vi "main_track.vi"(7 "camera notifier":refnum<notifier>, 8 "error in (no error)":errorcluster, 9 "tracking notifier in":refnum<notifier>, 10 "Median Filter Image":T2, 11 "Session In":T1) -> (0 "error out":errorcluster)   [LabVIEW 2019]
uses:
  <vilib>/vision/Image Controls.llb/IMAQ Image.ctl
  <vilib>/userdefined/High Color/IMAQdx.ctl
  CompletedTracksFunctionalGlobalOperations.ctl
  ActiveTracksFunctionalGlobalOperations.ctl
  <vilib>/vision/driver/IMAQdx.llb/IMAQdx Buffer Number Mode.ctl
  WormTrackSnippetCluster.ctl
  TrackTerminationReasonEnum.ctl
  <vilib>/Utility/error.llb/DialogType.ctl
  euclidean_distance_single.vi
  ParametersGlobal.vi
  DebugGlobal.vi
  StimulusObject.lvclass
  <vilib>/vision/NI_Vision_Development_Module.lvlib
  <vilib>/vision/driver/NI_Vision_Acquisition_Software.lvlib
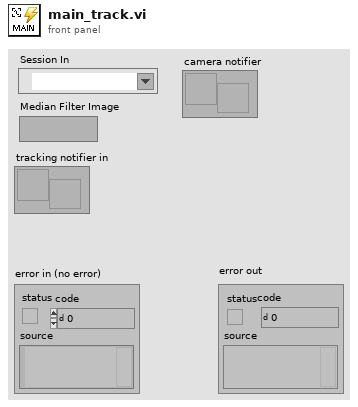
[diagram p1: front panel]
types:
  T1 = typedef "IMAQdx.ctl" = refnum<k21>
  T2 = typedef "IMAQ Image.ctl" = refnum<image>
  T3 = typedef "Particle Parameters" = i32
  T4 = cluster{"Measurement Parameter":T3, "Range Lower Value":dbl, "Range Upper Value":dbl, "Range":bool, "Measurement Type":bool}
  T5 = typedef "Image Type" = u32
  T6 = cluster{"Measurement Parameter":T3, "Range Lower Value":dbl, "Range Upper Value":dbl, "Range":bool, "Measurement Type":bool}[]
  T7 = typedef "NI_Vision_Acquisition_Software.lvlib/IMAQdx Buffer Number Mode.ctl" = enum32{"Next", "Last", "Buffer Number", "Every", "Last New"}
  T8 = typedef "ActiveTracksFunctionalGlobalOperations.ctl" = enum16{"Initialize", "ReadFullTrackGivenWormIndex", "WriteFullTrack", "ReadTrackSnippets", "WriteTrackGivenSnippets", "ReadStimulusSnippets", "StartNewTracksGivenSnippets", "EndTracksGivenSnippets", "WriteStimulusObjectGivenWormIndex", "CompleteAllActiveTracks", "ReturnAllActiveTrackIndecies"}
  T9 = typedef "CompletedTracksFunctionalGlobalOperations.ctl" = enum16{"Initialize", "ReturnAllTracks", "ReturnLastIndex", "SaveCompletedTracks", "TrimAndReturnAllTracks"}
  T10 = typedef "WormTrackSnippetCluster.ctl" = cluster{"Track Centroid Positions (Camera Pixel)":sgl[][], "Within Track Index":i32, "Camera Buffer Indecies":i32[], "Area (Camera Pixels)":i32, "Speed (mm/s)":sgl, "Direction (radians)":sgl, "Centerline Positions (Camera Pixel)":sgl[][], "Ellipse Ratio":sgl, "Termination Reason":T11, "Track Index":i32, "Bounding Rect Left":i32, "Bounding Rect Top":i32, "Bounding Rect Right":i32, "Bounding Rect Bottom":i32, "Mature Camera Buffer":i32, "Start Camera Buffer Index":i32, "Reverse Started Camera Buffer":i32}
  T11 = typedef "TrackTerminationReasonEnum.ctl" = enum16{"StillActive", "MaxDisplacement", "NoBlobsLeft", "AreaIncrease", "AreaDecrease", "ExperimentEnded"}
  T12 = typedef "WormTrackCluster.ctl" = cluster{"Track Centroid Positions (Camera Pixel)":sgl[][], "Within Track Index":i32, "Camera Buffer Indecies":i32[], "Area (Camera Pixels)":i32[], "Speed (mm/s)":sgl[], "Direction (radians)":sgl[], "Centerline Positions (Camera Pixel)":sgl[][][], "Ellipse Ratio":sgl[], "Stimulus Object":refnum<class "StimulusObject.lvclass">, "Termination Reason":T11, "Track Index":i32, "Mature Camera Buffer":i32, "Reverse Started Camera Buffer":i32}
  T13 = typedef "DialogType.ctl" = u16
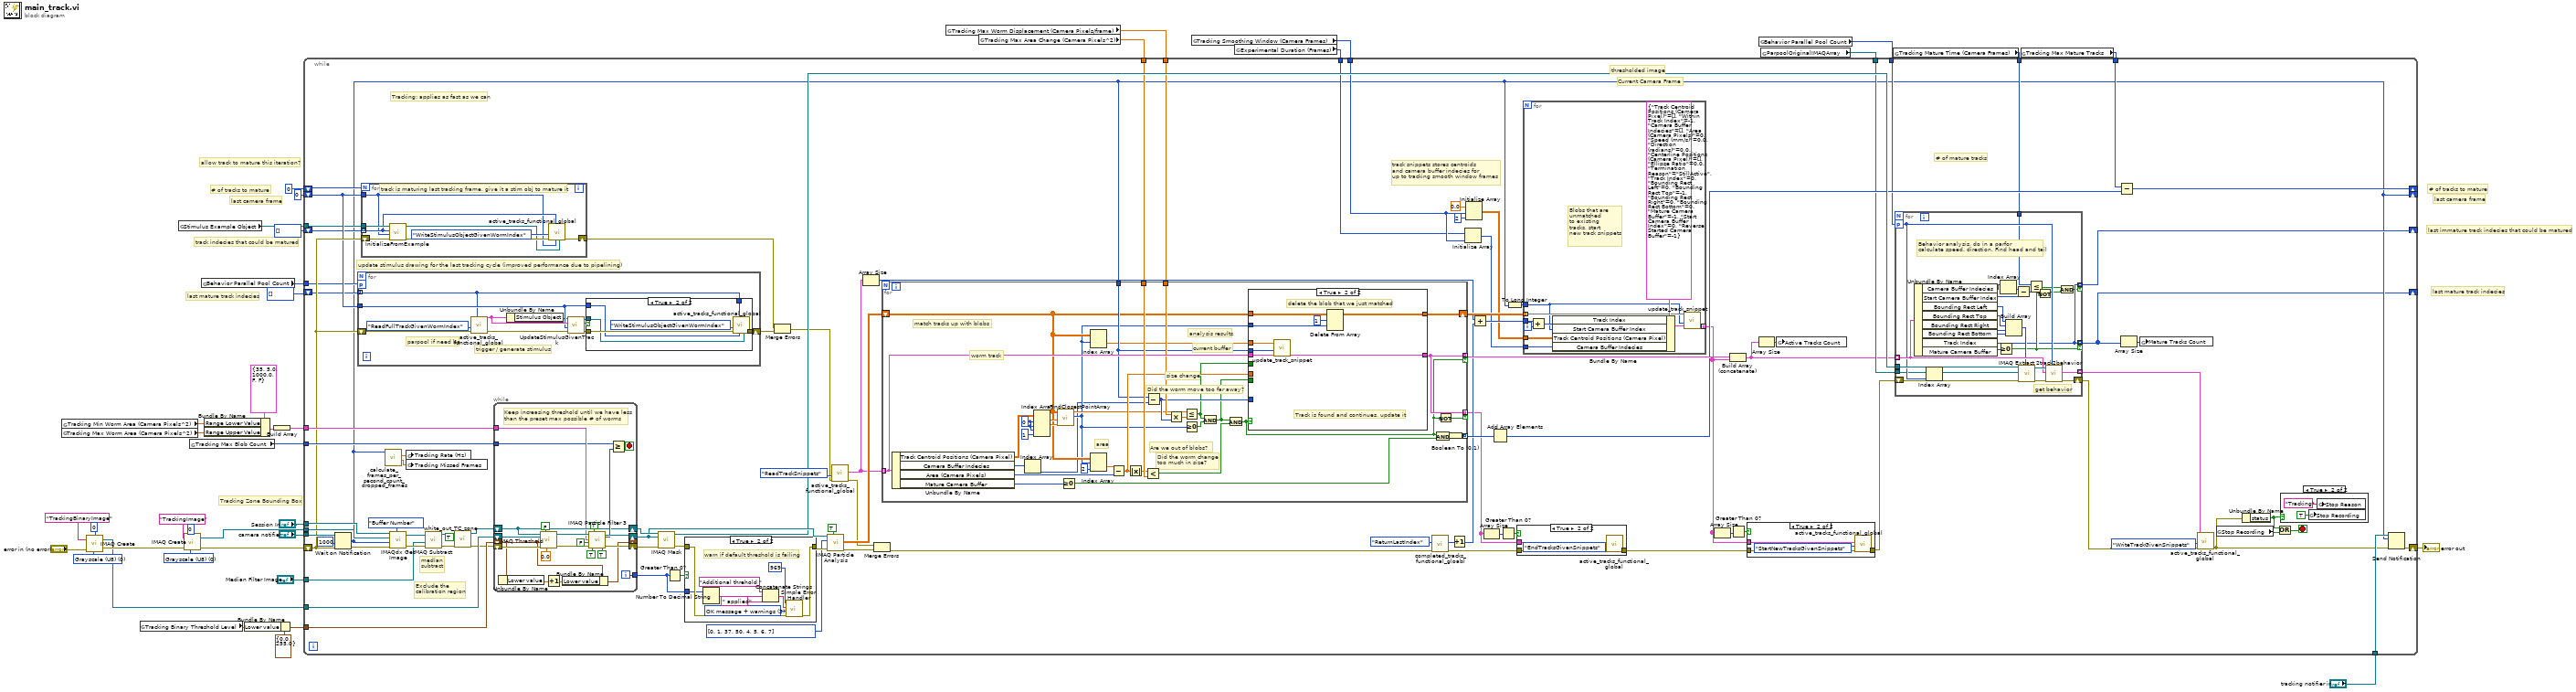
[diagram p0: block diagram]
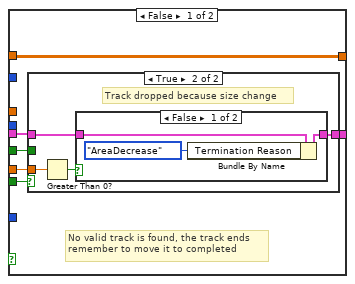
[diagram p6: hidden frame]
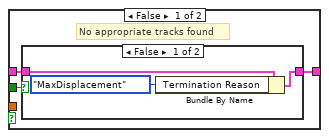
[diagram p7: hidden frame]
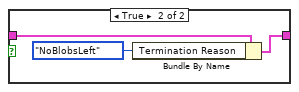
[diagram p8: hidden frame]
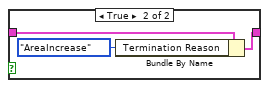
[diagram p9: hidden frame]
diagram:
  w35 = T5 0 items=["Grayscale (U8)", "Grayscale (I16)", "Grayscale (SGL)", "Complex (CSG)", "RGB (U32)", "HSL (U32)", "RGB (U64)", "Grayscale (U16)"] ("Image Type")
  w37 = T5 0 items=["Grayscale (U8)", "Grayscale (I16)", "Grayscale (SGL)", "Complex (CSG)", "RGB (U32)", "HSL (U32)", "RGB (U64)"] ("Image Type")
  # "allow track to mature this iteration?"
  # "last mature track indecies"
  # "track indecies that could be matured"
  # "last camera frame"
  # "# of tracks to mature"
  # "last mature track indecies"
  # "last immature track indecies that could be matured"
  # "last camera frame"
  # "# of tracks to mature"
  # "Tracking Zone Bounding Box"
  n1 = global read "ParametersGlobal.vi" "Tracking Max Worm Area (Camera Pixels^2)"() -> (w25:dbl)
  n2 = global read "ParametersGlobal.vi" "Tracking Min Worm Area (Camera Pixels^2)"() -> (w24:dbl)
  n3 = call "IMAQ Create"("Border Size"=0, "Image Name"="TrackingBinaryImage", "Image Type"=w35, "error in (no error)"="error in (no error)") -> ("New Image"=w30:T2, "error out"=w33:errorcluster)  [unwired: 1 in]
  n4 = global read "ParametersGlobal.vi" "Tracking Binary Threshold Level"() -> (w20:sgl)
  n5 = global read "ParametersGlobal.vi" "Stimulus Example Object"() -> (w1:refnum<class "StimulusObject.lvclass">)
  n6 = call "IMAQ Create"("Border Size"=0, "Image Name"="TrackingImage", "Image Type"=w37, "error in (no error)"=w33) -> ("New Image"=w28:T2, "error out"=w29:errorcluster)  [unwired: 1 in]
  n7 = global read "ParametersGlobal.vi" "Tracking Max Blob Count"() -> (w17:i32)
  n8 = global read "ParametersGlobal.vi" "Behavior Parallel Pool Count"() -> (w2:i32)
  n9 = Bundle By Name(cluster=T4 {"Measurement Parameter"=35, "Range Lower Value"=5.0, "Range Upper Value"=1000.0, "Range"=FALSE, "Measurement Type"=FALSE} ("Selection Value"), "Range Lower Value"=w24, "Range Upper Value"=w25) -> (w23:T4)
  n10 = Bundle By Name(cluster=cluster{"Lower value":sgl, "Upper value":sgl} {"Lower value"=0.0, "Upper value"=255.0} ("Range"), "Lower value"=w20) -> (w18:cluster{"Lower value":sgl, "Upper value":sgl})
  n11 = Build Array(w23) -> (w21:T6)
  n12 = global read "ParametersGlobal.vi" "Tracking Max Worm Displacement (Camera Pixels/frame)"() -> (w15:dbl)
  n13 = global read "ParametersGlobal.vi" "Tracking Max Area Change (Camera Pixels^2)"() -> (w16:dbl)
  n14 = global read "ParametersGlobal.vi" "Tracking Smoothing Window (Camera Frames)"() -> (w14:i32)
  n15 = global read "ParametersGlobal.vi" "Experimental Duration (Frames)"() -> (w13:i32)
  n16 = global read "ParametersGlobal.vi" "Behavior Parallel Pool Count"() -> (w12:i32)
  n17 = global read "ParametersGlobal.vi" "ParpoolOriginalIMAQArray"() -> (w10:T2[])
  n18 = global read "ParametersGlobal.vi" "Tracking Mature Time (Camera Frames)"() -> (w11:i32)
  n19 = global read "ParametersGlobal.vi" "Tracking Max Mature Tracks"() -> (w9:i16)
  n20 = while {
    tunnel: w28 -> [w88]
    tunnel: w30 -> [w45]
    shift-right: [w77] -> w39
    shift-left: w29 -> [w69]
    tunnel: "Median Filter Image" -> [w90]
    tunnel: "Session In" -> [w89]
    tunnel: w21 -> [w87]
    tunnel: w18 -> [w86]
    tunnel: w17 -> [w85]
    tunnel: w16 -> [w84]
    tunnel: w15 -> [w83]
    tunnel: w14 -> [w82]
    tunnel: w13 -> [w81]
    tunnel: w12 -> [w74]
    tunnel: w11 -> [w80]
    tunnel: w10 -> [w79]
    tunnel: w9 -> [w78]
    tunnel: "tracking notifier in" -> [w76]
    tunnel: "camera notifier" -> [w75]
    shift-right: [w73] -> _
    shift-left: i16 0 -> [w64]
    shift-right: [w58] -> _
    shift-left: u32 0 -> [w67]
    shift-right: [w72] -> _
    shift-left: i32[] [] -> [w66]
    shift-right: [w46] -> _
    shift-left: i32[] [] -> [w65]
    tunnel: w2 -> [w63]
    tunnel: w1 -> [w60]
    stop <- w98 stop-if-true
    w128 = T3[] [0, 1, 37, 50, 4, 5, 6, 7] items=["Center of Mass X", "Center of Mass Y", "First Pixel X", "First Pixel Y", "Bounding Rect Left", "Bounding Rect Top", "Bounding Rect Right", "Bounding Rect Bottom", "Max Feret Diameter Start X", "Max Feret Diameter Start Y", "Max Feret Diameter End X", "Max Feret Diameter End Y", "Max Horiz. Segment Length Left", "Max Horiz. Segment Length Right", "Max Horiz. Segment Length Row", "-", "Bounding Rect Width", "Bounding Rect Height", "Bounding Rect Diagonal", "Perimeter", "Convex Hull Perimeter", "Holes' Perimeter", "Max Feret Diameter", "Equivalent Ellipse Major Axis", "Equivalent Ellipse Minor Axis", "Equivalent Ellipse Minor Axis (Feret)", "Equivalent Rect Long Side", "Equivalent Rect Short Side", "Equivalent Rect Diagonal", "Equivalent Rect Short Side (Feret)", "Average Horiz. Segment Length", "Average Vert. Segment Length", "Hydraulic Radius", "Waddel Disk Diameter", "-", "Area", "Holes' Area", "Particle & Holes' Area", "Convex Hull Area", "Image Area", "-", "Number of Holes", "Number of Horiz. Segments", "Number of Vert. Segments", "-", "Orientation", "Max Feret Diameter Orientation", "-", "% Area/Image Area", "% Area/(Particle & Holes' Area)", "Ratio of Equivalent Ellipse Axes", "Ratio of Equivalent Rect Sides", "-", "Elongation Factor", "Compactness Factor", "Heywood Circularity Factor", "Type Factor", "-", "Sum X", "Sum Y", "Sum XX", "Sum XY", "Sum YY", "Sum XXX", "Sum XXY", "Sum XYY", "Sum YYY", "-", "Moment of Inertia XX", "Moment of Inertia XY", "Moment of Inertia YY", "Moment of Inertia XXX", "Moment of Inertia XXY", "Moment of Inertia XYY", "Moment of Inertia YYY", "Norm. Moment of Inertia XX", "Norm. Moment of Inertia XY", "Norm. Moment of Inertia YY", "Norm. Moment of Inertia XXX", "Norm. Moment of Inertia XXY", "Norm. Moment of Inertia XYY", "Norm. Moment of Inertia YYY", "Hu Moment 1", "Hu Moment 2", "Hu Moment 3", "Hu Moment 4", "Hu Moment 5", "Hu Moment 6", "Hu Moment 7"] ("Pixel Measurements")
    # "thresholded image"
    # "Current Camera Frame"
    # "update stimulus drawing for the last tracking cycle (improved performance due to pipelining)"
    # "Tracking: applies as fast as we can"
    # "median\nsubtract"
    # "track snippets stores centroids\nand camera buffer indecies for\nup to tracking smooth window frames"
    # "# of mature tracks"
    # "Exclude the\ncalibration region"
    n21 = Wait on Notification(notifier=w75, timeout in ms (-1)=1000, error in (no error)=w69) -> (notification=w58:u32, error out=w96:errorcluster)  [unwired: 1 in, 2 out]
    n22 = for {
      tunnel: w65 -> [w151] mode=indexing
      tunnel: w67 -> [w155]
      shift-right: [w156] -> w71
      shift-left: w69 -> [w157]
      workers-P: w63 -> [_]
      # "trigger / generate stimulus"
      # "parpool if need be"
      n23 = call "active_tracks_functional_global.vi"("Track Index In"=w151, "error in"=w157, "Operations"=ActiveTracksFunctionalGlobalOperations."ReadFullTrackGivenWormIndex") -> ("error out"=w160:errorcluster, "Full Worm Track Out"=w159:T12)  [unwired: 4 in, 3 out]
      n24 = Unbundle By Name(w159) -> ("Stimulus Object"=w154:refnum<class "StimulusObject.lvclass">)
      n25 = call-dynamic "UpdateStimulusGivenTrack.vi"("error in (no error)"=w160, "CameraFrame"=w155, "Track"=w159, "StimulusObject in"=w154) -> ("error out"=w158:errorcluster, "StimulusObject Changed"=w153:bool, "StimulusObject out"=w152:refnum<class "StimulusObject.lvclass">)  [unwired: 5 in]
      n26 = case shown="True" w153 {
        tunnel: w158 -> [w162 w168]
        tunnel: [w162 w166] -> w156
        tunnel: w155 -> [_ w165]
        tunnel: w152 -> [_ w164]
        tunnel: w151 -> [_ w163]
        frame False {
        }
        frame True {
          n27 = call "active_tracks_functional_global.vi"("StimulusObjectInput"=w164, "Camera Frame In"=w165, "Track Index In"=w163, "error in"=w168, "Operations"=ActiveTracksFunctionalGlobalOperations."WriteStimulusObjectGivenWormIndex") -> ("error out"=w166:errorcluster)  [unwired: 2 in, 4 out]
        }
      }
    }
    n28 = for {
      N: w64 -> [_]
      tunnel: w66 -> [w144] mode=indexing
      tunnel: w67 -> [w143]
      shift-right: [w148] -> w70
      shift-left: w69 -> [w147]
      tunnel: w60 -> [w146]
      # "track is maturing last tracking frame, give it a stim obj to mature it"
      n29 = call-dynamic "InitializeFromExample.vi"("error in (no error)"=w147, "StartingCameraFrame"=w143, "StimulusObjectIndex"=w144, "Stimulus in"=w146) -> ("error out"=w150:errorcluster, "Stimulus out"=w145:refnum<class "StimulusObject.lvclass">)  [unwired: 6 in]
      n30 = call "active_tracks_functional_global.vi"("StimulusObjectInput"=w145, "Camera Frame In"=w143, "Track Index In"=w144, "error in"=w150, "Operations"=ActiveTracksFunctionalGlobalOperations."WriteStimulusObjectGivenWormIndex") -> ("error out"=w148:errorcluster)  [unwired: 2 in, 4 out]
    }
    n31 = call "calculate_frames_per_second_count_dropped_frames.vi"("Buffer Number"=w58) -> ("Missed Frames"=w91:dbl, "Processed Frames/s"=w92:dbl)  [unwired: 8 in, 1 out]
    n32 = call <vilib>:"IMAQdx Get Image.vi"("Buffer Number Mode (Next)"=IMAQdx_Buffer_Number_Mode."Buffer Number", "error in"=w96, "Buffer Number In"=w58, "Image In"=w88, "Session In"=w89) -> ("error out"=w95:errorcluster, "Image Out"=w94:T2)  [unwired: 3 in, 2 out]
    n33 = global write "DebugGlobal.vi" "Tracking Rate (Hz)"(w92) -> ()
    n34 = global write "DebugGlobal.vi" "Tracking Missed Frames"(w91) -> ()
    n35 = call "IMAQ Subtract"("Image Src A"=w94, "Image Src B"=w90, "error in (no error)"=w95) -> ("Image Dst Out"=w42:T2, "error out"=w44:errorcluster)  [unwired: 4 in]
    n36 = call "white_out_TC_zone.vi"("error in (no error)"=w44, "Blackout?"=TRUE, "Refnum in"=w42) -> ("error out"=w43:errorcluster, "Refnum out"=w41:T2)  [unwired: 7 in]
    n37 = while {
      shift-right: [w296] -> _
      shift-left: w86 -> [w294]
      shift-right: [w302] -> w122
      shift-left: w45 -> [w286]
      shift-right: [w301] -> w125
      shift-left: w43 -> [w305]
      tunnel: [w300] -> w131
      shift-right: [w287] -> w123
      shift-left: w41 -> [w287]
      tunnel: w87 -> [w285]
      tunnel: w85 -> [w284]
      i -> [w300]
      stop <- w299 stop-if-true
      # "Keep increasing threshold until we have less\nthan the preset max possible # of worms"
      n38 = Unbundle By Name(w294) -> ("Lower value"=w298:sgl)
      n39 = call "IMAQ Threshold"("Replace Value"=sgl 0.0, "Keep/Replace Value (Replace)"=FALSE, "error in (no error)"=w305, "Range"=w294, "Image Dst"=w286, "Image Src"=w287) -> ("error out"=w303:errorcluster, "Image Dst Out"=w288:T2)  [unwired: 4 in]
      n40 = Increment(x=w298) -> (x+1=w297:sgl)
      n41 = Bundle By Name(cluster=w294, "Lower value"=w297) -> (w296:cluster{"Lower value":sgl, "Upper value":sgl})
      n42 = call "IMAQ Particle Filter 3"("Image Src"=w288, "Connectivity 4/8 (8)"=TRUE, "Selection Values"=w285, "Keep/Remove Particles (F)"=FALSE, "error in (no error)"=w303, "Reject Border? (F)"=TRUE, "Fill Holes? (F)"=TRUE) -> ("Image Dst Out"=w302:T2, "Number of Particles"=w295:i32, "error out"=w301:errorcluster)  [unwired: 6 in]
      n43 = Greater Or Equal?(x=w284, y=w295) -> (x >= y?=w299:bool)
    }
    n44 = call "IMAQ Mask"("error in (no error)"=w125, "Image Mask"=w122, "Image Src"=w123) -> ("error out"=w124:errorcluster, "Image Dst Out"=w121:T2)  [unwired: 2 in]
    n45 = Greater Than 0?(x=w131) -> (x > 0?=w132:bool)
    n46 = case shown="True" w132 {
      tunnel: w124 -> [w274 w283]
      tunnel: [w274 w282] -> w130
      tunnel: w131 -> [_ w279]
      frame False {
      }
      frame True {
        w281 = T13 3 items=["no dialog", "OK message", "continue or stop message", "OK message + warnings", "continue/stop + warnings"] ("type of dialog (OK msg:1)")
        # "warn if default threshold is failing"
        n47 = Number To Decimal String(number=w279) -> (decimal integer string=w277:string)  [unwired: 1 in]
        n48 = Concatenate Strings("Additional threhold " ("error source (\" \")"), w277, " applied") -> (w275:string)
        n49 = call <vilib>:"Simple Error Handler.vi"("error code (no error:0)"=969, "error source (\" \")"=w275, "type of dialog (OK msg:1)"=w281, "error in (no error)"=w283) -> ("error out"=w282:errorcluster)  [unwired: 1 in, 4 out]
      }
    }
    n50 = Merge Errors(w70, w71) -> (w68:errorcluster)
    n51 = call "IMAQ Particle Analysis"("Connectivity 4/8 (8)"=TRUE, "error in (no error)"=w130, "Pixel Measurements"=w128, "Image"=w122) -> ("error out"=w110:errorcluster, "Particle Measurements (Pixels)"=w129:dbl[][])  [unwired: 2 in, 4 out]
    n52 = call "active_tracks_functional_global.vi"("error in"=w68, "Operations"=ActiveTracksFunctionalGlobalOperations."ReadTrackSnippets") -> ("error out"=w109:errorcluster, "Track Snippets Out"=w111:T10[])  [unwired: 5 in, 3 out]
    n53 = Array Size(array=w111) -> (size(s)=w118:i32)
    n54 = Merge Errors(w109, w110) -> (w108:errorcluster)
    n55 = for {
      tunnel: w111 -> [w236] mode=indexing
      tunnel: w83 -> [w233]
      tunnel: w84 -> [w238]
      tunnel: w58 -> [w232]
      shift-right: [w230] -> w127
      shift-left: w129 -> [w221]
      tunnel: [w218] -> w119 mode=indexing if=w214
      tunnel: [w218] -> w57 mode=indexing if=w217
      tunnel: [w212] -> w117 mode=indexing
      w211 = 0 ("index (row)")
      # "match tracks up with blobs"
      # "analysis results"
      # "area"
      # "Are we out of blobs?"
      # "size change"
      # "worm track"
      # "current buffer"
      # "Did the worm move too far away?"
      # "Did the worm change\ntoo much in size?"
      n56 = Unbundle By Name(w236) -> ("Track Centroid Positions (Camera Pixel)"=w240:sgl[][], "Camera Buffer Indecies"=w208:i32[], "Area (Camera Pixels)"=w209:i32, "Mature Camera Buffer"=w216:i32)
      n57 = Index Array(array=w208) -> (element=w207:i32)  [unwired: 1 in]
      n58 = Index Array(array=w240, index (row) #1=w211, index (col) #1=w211, index (row) #2=w211, index (col) #2=1 ("disabled index (col)")) -> (element #1=w226:sgl, element #2=w225:sgl)
      n59 = call "FindClosestPointArray.vi"("Y"=w225, "X"=w226, "Particle Measurements (Pixels)"=w221) -> ("ShortestDistanceIndex"=w220:i32, "ShortestDistance"=w229:sgl)  [unwired: 7 in]
      n60 = Greater Or Equal To 0?(x=w216) -> (x >= 0?=w215:bool)
      n61 = Index Array(array=w221, index (row)=w220) -> (element=w219:dbl[])  [unwired: 1 in]
      n62 = Index Array(array=w221, index (row)=w220, index (col)=2 ("disabled index (col)")) -> (element=w223:dbl)
      n63 = Subtract(x=w223, y=w209) -> (x-y=w234:dbl)
      n64 = Absolute Value(x=w234) -> (abs(x)=w235:dbl)
      n65 = Less?(x=w235, y=w238) -> (x < y?=w237:bool)
      n66 = Subtract(x=w232, y=w207) -> (x-y=w231:u32)
      n67 = Multiply(x=w233, y=w231) -> (x*y=w228:dbl)
      n68 = Less Or Equal?(x=w229, y=w228) -> (x <= y?=w224:bool)
      n69 = Greater Or Equal To 0?(x=w220) -> (x >= 0?=w239:bool)
      n70 = And(x=w224, y=w239) -> (x .and. y?=w227:bool)
      n71 = And(x=w227, y=w237) -> (x .and. y?=w214:bool)
      n72 = case shown="True" w214 {
        tunnel: w227 -> [w242 _]
        tunnel: w236 -> [w246 w269]
        tunnel: w234 -> [w245 _]
        tunnel: w232 -> [_ w267]
        tunnel: w231 -> [_ _]
        tunnel: [w244 w268] -> w218
        tunnel: w221 -> [w243 w273]
        tunnel: w220 -> [_ w271]
        tunnel: [w243 w270] -> w230
        tunnel: w224 -> [w241 _]
        tunnel: w219 -> [_ w266]
        frame False {
          # "No valid track is found, the track ends\nremember to move it to completed"
          n73 = case shown="True" w242 {
            tunnel: w246 -> [w249 w257]
            tunnel: [w248 w256] -> w244
            tunnel: w245 -> [_ w259]
            tunnel: w241 -> [w247 _]
            frame False {
              # "No appropriate tracks found"
              n74 = case shown="False" w247 {
                tunnel: w249 -> [w252 w255]
                tunnel: [w251 w254] -> w248
                frame False {
                  n75 = Bundle By Name(cluster=w252, "Termination Reason"=TrackTerminationReasonEnum."MaxDisplacement") -> (w251:T10)
                }
                frame True {
                  n76 = Bundle By Name(cluster=w255, "Termination Reason"=TrackTerminationReasonEnum."NoBlobsLeft") -> (w254:T10)
                }
              }
            }
            frame True {
              # "Track dropped because size change"
              n77 = Greater Than 0?(x=w259) -> (x > 0?=w258:bool)
              n78 = case shown="False" w258 {
                tunnel: w257 -> [w262 w265]
                tunnel: [w261 w264] -> w256
                frame False {
                  n79 = Bundle By Name(cluster=w262, "Termination Reason"=TrackTerminationReasonEnum."AreaDecrease") -> (w261:T10)
                }
                frame True {
                  n80 = Bundle By Name(cluster=w265, "Termination Reason"=TrackTerminationReasonEnum."AreaIncrease") -> (w264:T10)
                }
              }
            }
          }
        }
        frame True {
          # "delete the blob that we just matched"
          # "Track is found and continues, update it"
          n81 = call "update_track_snippet.vi"("Input Track Snippet"=w269, "Current Camera Buffer Number"=w267, "Particle Analysis Output"=w266) -> ("Output Track Snippet"=w268:T10)  [unwired: 8 in]
          n82 = Delete From Array(array=w273, length=1, index (row)=w271) -> (array with subset deleted=w270:dbl[][])  [unwired: 1 in, 1 out]
        }
      }
      n83 = And(x=w214, y=w215) -> (x .and. y?=w213:bool)
      n84 = Not(x=w214) -> (.not. x?=w217:bool)
      n85 = Boolean To (0,1)(Boolean=w213) -> (0, 1=w212:i16)
    }
    n86 = call "completed_tracks_functional_gloabl.vi"("error in (no error)"=w108, 10:CompletedTracksFunctionalGlobalOperations."ReturnLastIndex") -> ("error out"=w107:errorcluster, "LastTrackIndex"=w113:i32)  [unwired: 6 in, 2 out]
    n87 = Increment(x=w113) -> (x+1=w114:i32)
    n88 = Initialize Array(w81, w82) -> (w101:i32[])
    n89 = Initialize Array(sgl 0.0 ("Numeric"), w82, 2 ("dimension size")) -> (w102:sgl[][])
    n90 = Add(x=w118, y=w114) -> (x+y=w126:i32)
    n91 = Array Size(array=w57) -> (size(s)=w56:i32)
    n92 = Add Array Elements(numeric array=w117) -> (sum=w116:i16)
    n93 = Greater Than 0?(x=w56) -> (x > 0?=w55:bool)
    n94 = To Long Integer(number=w58) -> (32bit integer=w59:i32)
    n95 = case shown="True" w55 {
      tunnel: w107 -> [w138 w141]
      tunnel: [w138 w140] -> w54
      tunnel: w57 -> [_ w139]
      frame False {
      }
      frame True {
        n96 = call "active_tracks_functional_global.vi"("error in"=w141, "Operations"=ActiveTracksFunctionalGlobalOperations."EndTracksGivenSnippets", "Track Snippets In"=w139) -> ("error out"=w140:errorcluster)  [unwired: 4 in, 4 out]
      }
    }
    n97 = for {
      tunnel: w127 -> [w204] mode=indexing
      tunnel: [w206] -> w52 mode=indexing
      tunnel: w126 -> [w201]
      tunnel: w59 -> [w199]
      tunnel: w102 -> [w198]
      tunnel: w101 -> [w197]
      i -> [w200]
      # "Blobs that are\nunmatched\nto existing \ntracks, start \nnew track snippets"
      n98 = Add(x=w201, y=w200) -> (x+y=w202:i32)
      n99 = Bundle By Name(cluster=T10 {"Track Centroid Positions (Camera Pixel)"=[], "Within Track Index"=-1, "Camera Buffer Indecies"=[], "Area (Camera Pixels)"=0, "Speed (mm/s)"=0.0, "Direction (radians)"=0.0, "Centerline Positions (Camera Pixel)"=[], "Ellipse Ratio"=0.0, "Termination Reason"=enum."StillActive", "Track Index"=0, "Bounding Rect Left"=0, "Bounding Rect Top"=-1, "Bounding Rect Right"=0, "Bounding Rect Bottom"=0, "Mature Camera Buffer"=-1, "Start Camera Buffer Index"=0, "Reverse Started Camera Buffer"=-1} ("Track Snippet"), "Track Index"=w202, "Start Camera Buffer Index"=w199, "Track Centroid Positions (Camera Pixel)"=w198, "Camera Buffer Indecies"=w197) -> (w203:T10)
      n100 = call "update_track_snippet.vi"("Input Track Snippet"=w203, "Current Camera Buffer Number"=w199, "Particle Analysis Output"=w204) -> ("Output Track Snippet"=w206:T10)  [unwired: 8 in]
    }
    n101 = Array Size(array=w52) -> (size(s)=w53:i32)
    n102 = Build Array (concatenate)(w119, w52) -> (w61:T10[])
    n103 = Greater Than 0?(x=w53) -> (x > 0?=w51:bool)
    n104 = case shown="True" w51 {
      tunnel: w52 -> [_ w136]
      tunnel: [w133 w135] -> w49
      tunnel: w54 -> [w133 w134]
      frame False {
      }
      frame True {
        n105 = call "active_tracks_functional_global.vi"("error in"=w134, "Operations"=ActiveTracksFunctionalGlobalOperations."StartNewTracksGivenSnippets", "Track Snippets In"=w136) -> ("error out"=w135:errorcluster)  [unwired: 4 in, 4 out]
      }
    }
    n106 = Array Size(array=w61) -> (size(s)=w62:i32)
    n107 = global write "DebugGlobal.vi" "Active Tracks Count"(w62) -> ()
    n108 = for {
      tunnel: w61 -> [w192] mode=indexing
      tunnel: w121 -> [w195]
      tunnel: [w185] -> w105 mode=indexing
      workers-P: w74 -> [w186]
      tunnel: [w178] -> w46 mode=indexing if=w180
      tunnel: [w178] -> w72 mode=indexing if=w177
      tunnel: w80 -> [w174]
      tunnel: w79 -> [w173]
      shift-right: [w171] -> w48
      shift-left: w49 -> [w172]
      # "get behavior"
      # "Behavior analysis, do in a parfor\ncalculate speed, direction. Find head and tail"
      n109 = Unbundle By Name(w192) -> ("Camera Buffer Indecies"=w176:i32[], "Start Camera Buffer Index"=w183:i32, "Bounding Rect Left"=w191:i32, "Bounding Rect Top"=w190:i32, "Bounding Rect Right"=w189:i32, "Bounding Rect Bottom"=w188:i32, "Track Index"=w178:i32, "Mature Camera Buffer"=w184:i32)
      n110 = Index Array(array=w173, index=w186) -> (element=w196:T2)
      n111 = Greater Or Equal To 0?(x=w184) -> (x >= 0?=w180:bool)
      n112 = Index Array(array=w176) -> (element=w175:i32)  [unwired: 1 in]
      n113 = Build Array(w191, w190, w189, w188) -> (w187:i32[])
      n114 = Subtract(x=w175, y=w183) -> (x-y=w182:i32)
      n115 = call "IMAQ Extract 2"("Optional Rectangle"=w187, "error in (no error)"=w172, "Image Dst"=w196, "Image Src"=w195) -> ("error out"=w194:errorcluster, "Image Dst Out"=w193:T2)  [unwired: 6 in]
      n116 = Less Or Equal?(x=w174, y=w182) -> (x <= y?=w181:bool)
      n117 = Not(x=w180) -> (.not. x?=w179:bool)
      n118 = call "track2behavior.vi"("ParallelPoolID"=w186, "error in (no error)"=w194, "Track In"=w192, "Original Worm Image"=w193) -> ("error out"=w171:errorcluster, "Track Out"=w185:T10)  [unwired: 6 in]
      n119 = And(x=w181, y=w179) -> (x .and. y?=w177:bool)
    }
    n120 = Subtract(x=w78, y=w116) -> (x-y=w73:i16)
    n121 = Array Size(array=w46) -> (size(s)=w47:i32)
    n122 = global write "DebugGlobal.vi" "Mature Tracks Count"(w47) -> ()
    n123 = call "active_tracks_functional_global.vi"("error in"=w48, "Operations"=ActiveTracksFunctionalGlobalOperations."WriteTrackGivenSnippets", "Track Snippets In"=w105) -> ("error out"=w50:errorcluster)  [unwired: 4 in, 4 out]
    n124 = global read "DebugGlobal.vi" "Stop Recording"() -> (w99:bool)
    n125 = Unbundle By Name(w50) -> ("status"=w100:bool)
    n126 = Or(x=w100, y=w99) -> (x .or. y?=w98:bool)
    n127 = case shown="True" w100 {
      frame False {
      }
      frame True {
        n128 = global write "DebugGlobal.vi" "Stop Recording"(TRUE ("stop")) -> ()
        n129 = global write "DebugGlobal.vi" "Stop Reason"("Tracking" ("Stop Debug")) -> ()
      }
    }
    n130 = Send Notification(notification=w58, notifier=w76, error in (no error)=w50) -> (error out=w77:errorcluster)  [unwired: 1 out]
  }
  "error out" <- w39
